vi "NTPlayer.vi"() -> ()   [LabVIEW 2023]
panel:
  out "Waveform Chart":i64[][](graph)
  in  "stop":bool
  out "appended array":string[](array[string])
  out "Deviation by row":i64[][](array[numeric])
  out "Average in row":u64[](array[numeric]) format="%-2.0f"
  in  "Deviation":bool
  in  "Settings Button":bool
  in  "Stop Button":bool
  out "?":string[][](array[string])
  out "Boolean":bool
  in  "Check":bool
  in  "Play":bool
  in  "Last Draw":i64[](array[numeric])
  out "Matches":i64[][](array[numeric])
  out "Matches":i32[](array[numeric])
  out "Your Suppose":i32[][](array[numeric])
  # "Deviation"
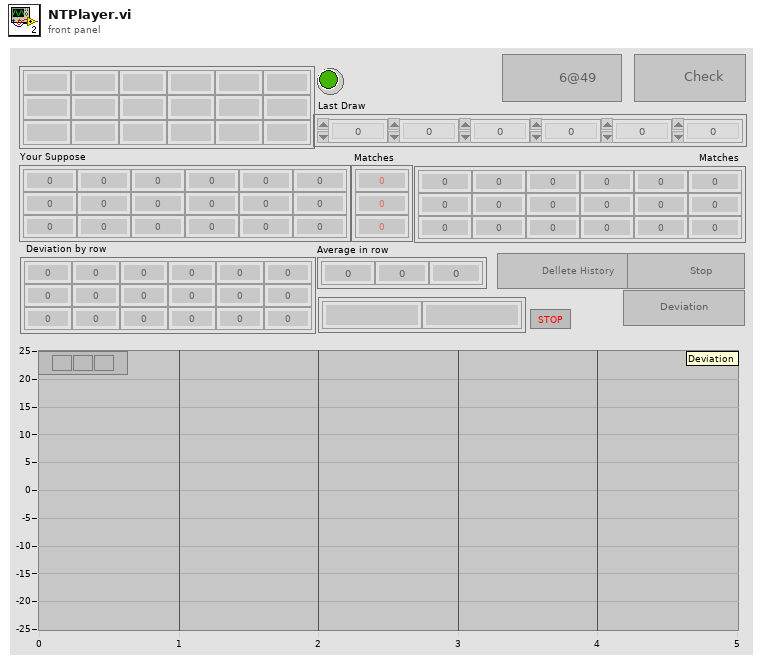
[diagram p1: front panel]
types:
  T1 = enum8{"Enabled", "Disabled", "Disabled and Grayed Out"}
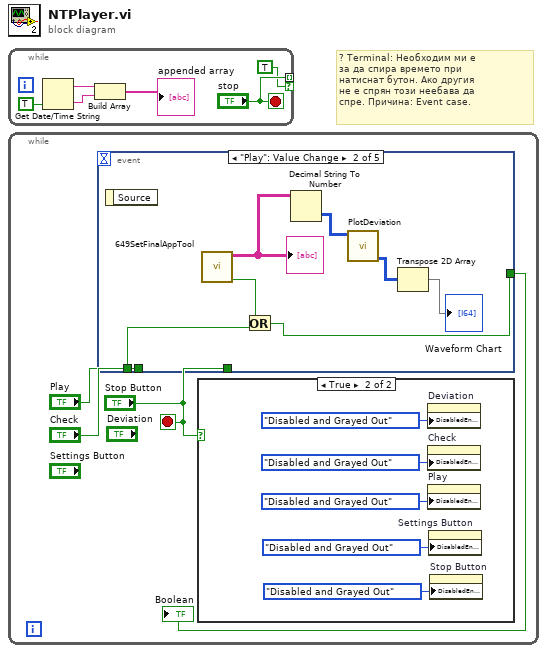
[diagram p0: block diagram]
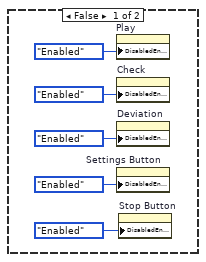
[diagram p2: hidden frame]
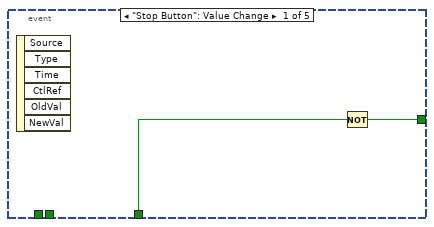
[diagram p3: hidden frame]
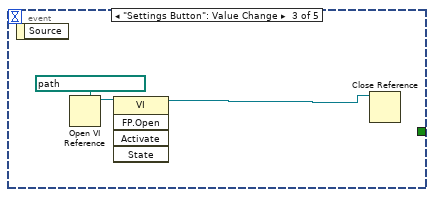
[diagram p4: hidden frame]
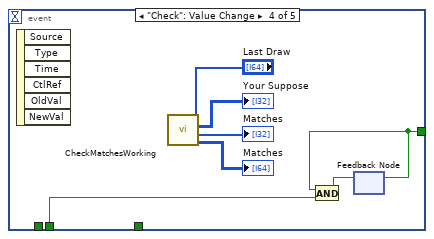
[diagram p5: hidden frame]
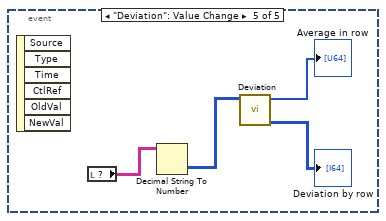
[diagram p6: hidden frame]
diagram:
  # "? Terminal: Необходим ми е\nза да спира времето при \nнатиснат бутон. Ако другия \nне е спрян този неебава да\nспре. Причина: Event case."
  n1 = while {
    tunnel: ["stop"] -> _ mode=indexing if=TRUE
    stop <- "stop" stop-if-true
    n2 = Get Date/Time String(want seconds? (F)=TRUE) -> (date string=w4:string, time string=w6:string)  [unwired: 2 in]
    n3 = Build Array(w4, w6) -> (→"appended array":string[])
  }
  n4 = while {
    stop <- "Stop Button" stop-if-true
    n5 = event shown="[1] \"Play\": Value Change" {
      selector: _ -> [_ _ _ _ _]
      dyn-events: _ -> [_ _ _ _ _]
      timeout: _ -> [_ _ _ _ _]
      tunnel: [w22 w27 _ w33 _] -> w10
      tunnel: "Check" -> [_ _ _ w35 _]
      tunnel: "Play" -> [_ w28 _ _ _]
      tunnel: "Stop Button" -> [w21 _ _ _ _]
      event "Stop Button": Value Change {
        n6 = event-data() -> ()  [unwired: 1 in, 6 out]
        n7 = Not(x=w21) -> (.not. x?=w22:bool)
      }
      event "Play": Value Change {
        n8 = event-data() -> ()  [unwired: 1 in, 1 out]
        n9 = call "649SetFinalAppTool.vi"() -> ("Out Arr"=w26:string[][], "Boolean"=w29:bool)  [unwired: 8 in, 1 out]
        "?" <- w26
        n10 = Or(x=w29, y=w28) -> (x .or. y?=w27:bool)
        n11 = Decimal String To Number(string=w26) -> (number=w25:i32[][])  [unwired: 2 in, 1 out]
        n12 = call "PlotDeviation.vi"("Array"=w25) -> ("Deviation by row"=w24:i64[][])  [unwired: 8 in, 2 out]
        n13 = Transpose 2D Array(2D array=w24) -> (transposed array=→"Waveform Chart":i64[][])
      }
      event "Settings Button": Value Change {
        n14 = event-data() -> ()  [unwired: 1 in, 1 out]
        n15 = Open VI Reference(vi path=path "/Users/blagojnikolov/Library/Mobile Documents/com~apple~CloudDocs/» LabView/LabView/Project'24/Projects/649/PlotDeviation.vi") -> (vi reference=w31:refnum<vi>)  [unwired: 5 in, 1 out]
        n16 = invoke class="VI" method="FP.Open"(reference=w31) -> (reference out=w30:refnum<vi>)  [unwired: 4 in, 4 out]
        n17 = Close Reference(reference=w30) -> ()  [unwired: 1 in, 1 out]
      }
      event "Check": Value Change {
        n18 = event-data() -> ()  [unwired: 1 in, 6 out]
        n19 = call "CheckMatchesWorking.vi"("Последен тираж"="Last Draw") -> (0:→"Matches":i64[][], "Съвпадения"=→"Matches":i32[], "Залози"=→"Your Suppose":i32[][])  [unwired: 8 in]
        n20 = feedback #1() -> (w33:bool)  [unwired: 1 in]
        n21 = And(x=w33, y=w35) -> (x .and. y?=w34:bool)
        n22 = feedback-in #1(w34) -> ()
      }
      event "Deviation": Value Change {
        n23 = event-data() -> ()  [unwired: 1 in, 6 out]
        n24 = local read item#8() -> (w41:string[][])
        n25 = Decimal String To Number(string=w41) -> (number=w40:i32[][])  [unwired: 2 in, 1 out]
        n26 = call "Deviation.vi"("2D  Array"=w40) -> ("Deviation by row"=→"Deviation by row":i64[][], "Average in row"=→"Average in row":u64[])  [unwired: 9 in]
      }
    }
    "Boolean" <- w10
    n27 = case shown="True" "Stop Button" {
      frame False {
        n28 = property on="Play" class="Bool"("DisabledEnum"=T1."Enabled" ("Disabled")) -> ()  [unwired: 2 in, 2 out]
        n29 = property on="Check" class="Bool"("DisabledEnum"=T1."Enabled" ("Disabled")) -> ()  [unwired: 2 in, 2 out]
        n30 = property on="Deviation" class="Bool"("DisabledEnum"=T1."Enabled" ("Disabled")) -> ()  [unwired: 2 in, 2 out]
        n31 = property on="Settings Button" class="Bool"("DisabledEnum"=T1."Enabled" ("Disabled")) -> ()  [unwired: 2 in, 2 out]
        n32 = property on="Stop Button" class="Bool (strict)"("DisabledEnum"=T1."Enabled" ("Disabled")) -> ()  [unwired: 2 in, 2 out]
      }
      frame True {
        n33 = property on="Deviation" class="Bool"("DisabledEnum"=T1."Disabled and Grayed Out" ("Disabled")) -> ()  [unwired: 2 in, 2 out]
        n34 = property on="Check" class="Bool"("DisabledEnum"=T1."Disabled and Grayed Out" ("Disabled")) -> ()  [unwired: 2 in, 2 out]
        n35 = property on="Play" class="Bool"("DisabledEnum"=T1."Disabled and Grayed Out" ("Disabled")) -> ()  [unwired: 2 in, 2 out]
        n36 = property on="Settings Button" class="Bool"("DisabledEnum"=T1."Disabled and Grayed Out" ("Disabled")) -> ()  [unwired: 2 in, 2 out]
        n37 = property on="Stop Button" class="Bool (strict)"("DisabledEnum"=T1."Disabled and Grayed Out" ("Disabled")) -> ()  [unwired: 2 in, 2 out]
      }
    }
  }
